vi "DD_CloseRef_TS_Step.vi"(0 "Engine Reference":refnum<k7>, 1 "Precondition":string, 5 "Sequence File Ref":refnum<k7>, 7 "Step Name":string="Close DIAdem Ref", 9 "Requirement":string, 11 "error in":errorcluster, 12 "index":i32) -> (4 "Engine reference(out)":refnum<k7>, 6 "Sequence File Ref(out)":refnum<k7>, 15 "error out":errorcluster)   [LabVIEW 2010]
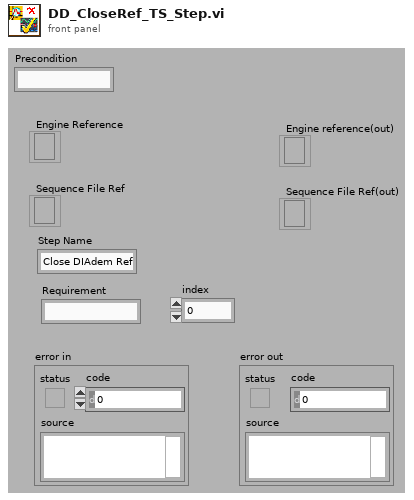
[diagram p1: front panel]
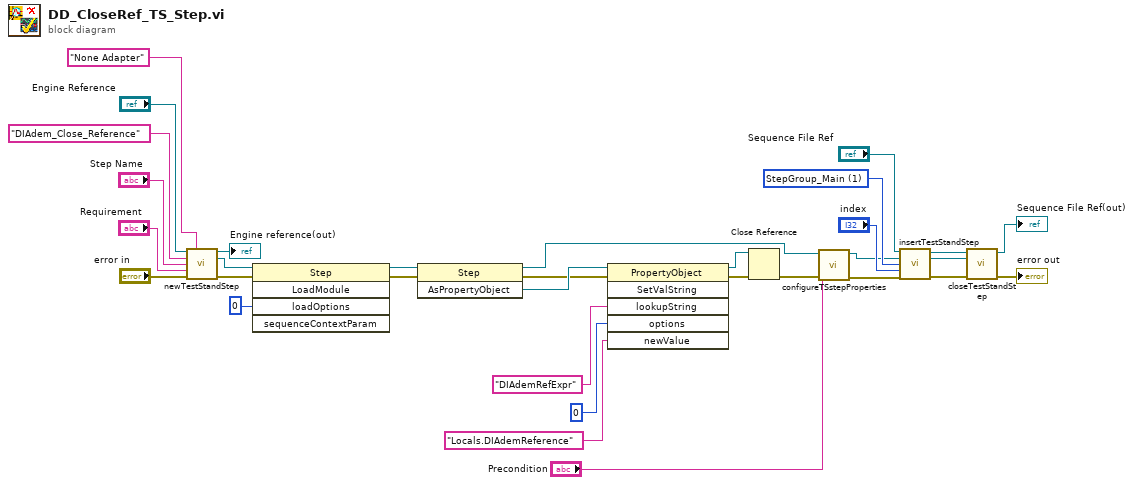
[diagram p0: block diagram]
diagram:
  w21 = 1 items=["StepGroup_Setup", "StepGroup_Main", "StepGroup_Cleanup"] ("Step Group")
  n1 = call "newTestStandStep.vi"("Engine reference"="Engine Reference", "adapterKeyNameVal"="None Adapter", "stepType"="DIAdem_Close_Reference", "Step Name"="Step Name", "Requirement"="Requirement", "error in"="error in") -> ("Engine reference(out)"=→"Engine reference(out)":refnum<k7>, "NewStep (out)"=w18:refnum<k7>, "error out"=w19:errorcluster)  [unwired: 7 in]
  n2 = invoke class="Step" method="LoadModule"(reference=w18, error in=w19, "loadOptions"=0) -> (reference out=w26:refnum<k7>, error out=w27:errorcluster)  [unwired: 2 in, 3 out]
  n3 = invoke class="Step" method="AsPropertyObject"(reference=w26, error in=w27) -> (reference out=w2:refnum<k7>, error out=w9:errorcluster, "AsPropertyObject"=w10:refnum<k7>)  [unwired: 1 in]
  n4 = invoke class="PropertyObject" method="SetValString"(reference=w10, error in=w9, "lookupString"="DIAdemRefExpr", "options"=0, "newValue"="Locals.DIAdemReference") -> (reference out=w32:refnum<k7>, error out=w31:errorcluster)  [unwired: 1 in, 4 out]
  n5 = Close Reference(reference=w32, error in (no error)=w31) -> (error out=w5:errorcluster)
  n6 = call "configureTSstepProperties.vi"("error in"=w5, "Precondition"="Precondition", "NewStep (in)"=w2) -> ("error out"=w4:errorcluster, "NewStep (out)"=w3:refnum<k7>)  [unwired: 7 in]
  n7 = call "insertTestStandStep.vi"("Sequence File Ref"="Sequence File Ref", "Step to insert"=w3, "Step Group"=w21, "index"="index", "error out"=w4) -> ("Sequence File Ref(out)"=w8:refnum<k7>, "Step to insert (out)"=w7:refnum<k7>, "error out"=w23:errorcluster)  [unwired: 8 in]
  n8 = call "closeTestStandStep.vi"("error in"=w23, "NewStep"=w7, "Sequence File Ref"=w8) -> ("error out"=→"error out":errorcluster, "Sequence File Ref(out)"=→"Sequence File Ref(out)":refnum<k7>)  [unwired: 7 in]
